vi "Write Processor.vi"(8 "error in":errorcluster, 10 "Processor":i32=-2, 11 "Standard Engine Repo Data in":refnum<class "Standard Engine Configuration.lvclass">) -> (0 "error out":errorcluster, 3 "Standard Engine Repo Data out":refnum<class "Standard Engine Configuration.lvclass">)   [LabVIEW 2013, in "Standard Engine Configuration.lvclass"]
doc: "Specifies which CPU core the engine will execute on. Use the value of '-2' to indicate that the engine may run on any core."
uses:
  Standard Engine Configuration.lvclass
  Standard Engine Configuration.lvclass/Standard Engine Configuration.ctl
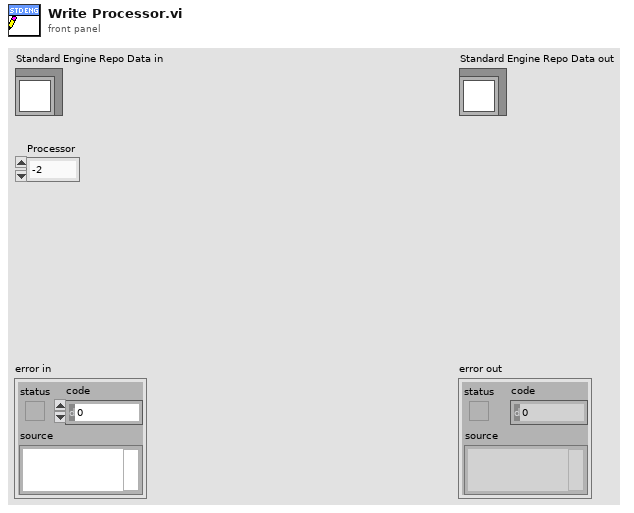
[diagram p1: front panel]
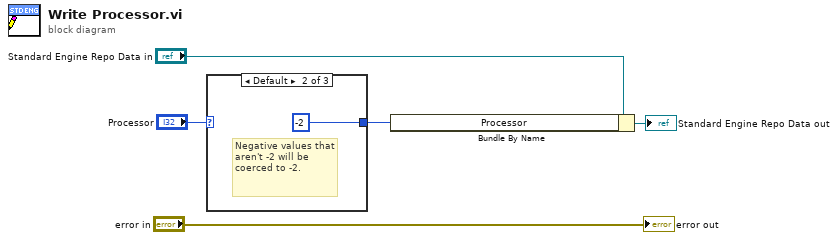
[diagram p0: block diagram]
diagram:
  n1 = case shown="Default" "Processor" {
    selector: "Processor" -> [w6 _ w8]
    tunnel: [w6 -2 ("Processor") w8] -> w1
    frame 0.. {
    }
    frame Default {
      # "Negative values that aren't -2 will be coerced to -2."
    }
    frame -2 {
    }
  }
  n2 = Bundle By Name(cluster="Standard Engine Repo Data in", "Processor"=w1) -> (→"Standard Engine Repo Data out":refnum<class "Standard Engine Configuration.lvclass">)
  "error out" <- "error in"
